vi "niFPGA BW CU Order 4 (32-bit).vi"(0 "filter state in":T1, 1 "reset":bool, 5 "input data":i32, 7 "accumulator in":fxp<+/-,36,32>, 9 "adder in":fxp<+/-,34,34>, 11 "iteration":u8, 12 "In shift":i8=-1, 13 "lowpass?":bool) -> (4 "filter state out":T1, 6 "state to multiply":i32, 8 "accumulator out":fxp<+/-,36,32> format="%.14g", 10 "adder out":fxp<+/-,34,34>, 15 "terminate":bool)   [LabVIEW 2017]
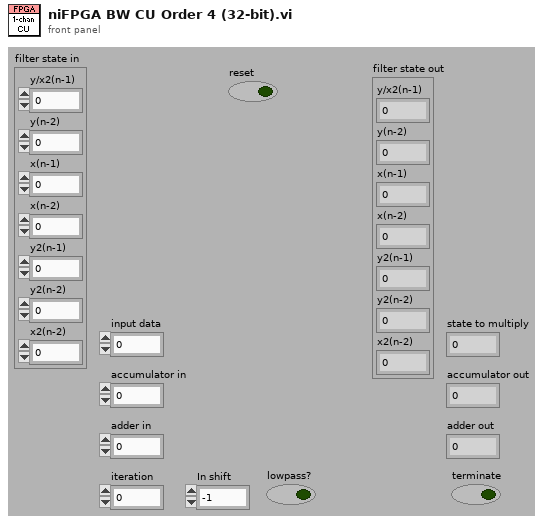
[diagram p1: front panel]
types:
  T1 = cluster{"y/x2(n-1)":i32, "y(n-2)":i32, "x(n-1)":i32, "x(n-2)":i32, "y2(n-1)":i32, "y2(n-2)":i32, "x2(n-2)":i32}
  T2 = cluster{"y(n)=x(n) 2":i32, "y(n-2)":i32, "x(n-1)":i32, "x(n-2)":i32, "y(n-1) 2":i32, "y(n-2) 2":i32, "x(n-2) 2":i32}
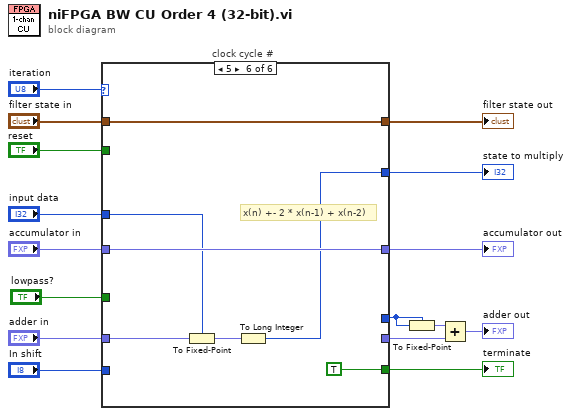
[diagram p0: block diagram]
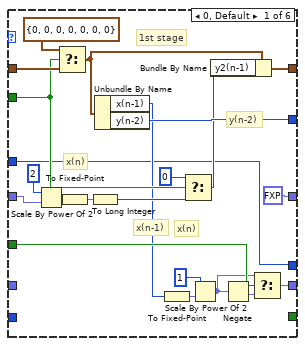
[diagram p2: hidden frame]
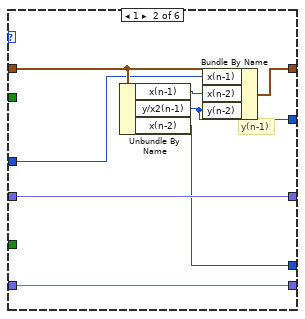
[diagram p3: hidden frame]
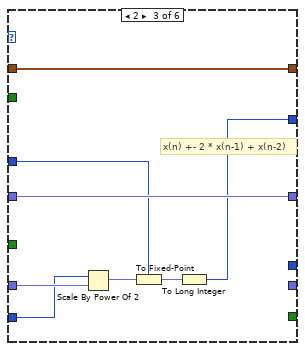
[diagram p4: hidden frame]
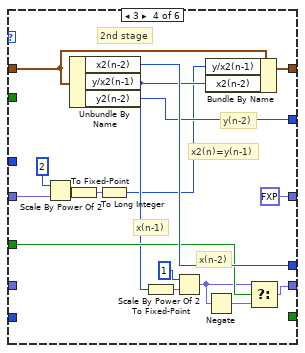
[diagram p5: hidden frame]
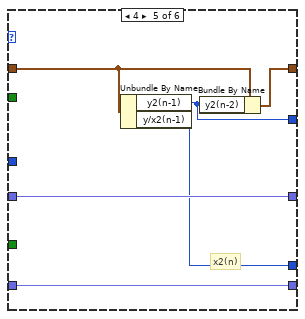
[diagram p6: hidden frame]
diagram:
  n1 = case "clock cycle #" shown="5" "iteration" {
    tunnel: [w38 w42 w53 w71 w73 w82] -> w3
    tunnel: "input data" -> [w17 w41 w47 _ _ w78]
    tunnel: [w28 w46 _ w61 w77 _] -> w10
    tunnel: "adder in" -> [_ w46 w50 _ w77 w80]
    tunnel: [w36 w44 w49 w69 w75 w81] -> w12
    tunnel: [w17 w39 _ w70 w72 _] -> w2
    tunnel: [fxp<+/-,36,32> 0.0 ("Numeric") w45 w54 fxp<+/-,36,32> 0.0 ("accumulator in") w76 w83] -> w11
    tunnel: [_ _ _ _ _ TRUE] -> w9
    tunnel: "reset" -> [w31 _ _ _ _ _]
    tunnel: "accumulator in" -> [w25 w45 w54 w60 w76 w83]
    tunnel: "filter state in" -> [w32 w43 w53 w66 w74 w82]
    tunnel: "In shift" -> [_ _ w48 _ _ _]
    tunnel: "lowpass?" -> [w29 _ _ w67 _ _]
    frame 0, Default {
      # "1st stage"
      # "x(n)"
      # "x(n)"
      # "x(n-1)"
      # "y(n-2)"
      n2 = Scale By Power Of 2(n=2, x=w25) -> (x*2^n=w26:fxp<+/-,36,32>)
      n3 = Select(t=T2 {"y(n)=x(n) 2"=0, "y(n-2)"=0, "x(n-1)"=0, "x(n-2)"=0, "y(n-1) 2"=0, "y(n-2) 2"=0, "x(n-2) 2"=0} ("output cluster"), s=w31, f=w32) -> (s? t:f=w34:T1)
      n4 = To Fixed-Point(number=w26) -> (fixed-point=w27:fxp<+/-,32,32>)  [unwired: 1 out]
      n5 = To Long Integer(number=w27) -> (32bit integer=w23:i32)
      n6 = Unbundle By Name(w34) -> ("x(n-1)"=w19:i32, "y(n-2)"=w36:i32)
      n7 = To Fixed-Point(number=w19) -> (fixed-point=w21:fxp<+/-,33,33>)  [unwired: 1 out]
      n8 = Select(t=0, s=w31, f=w23) -> (s? t:f=w22:i32)
      n9 = Scale By Power Of 2(n=1, x=w21) -> (x*2^n=w18:fxp<+/-,33,33>)
      n10 = Bundle By Name(cluster=w34, "y2(n-1)"=w22) -> (w38:T1)
      n11 = Negate(x=w18) -> (-x=w30:fxp<+/-,34,34>)
      n12 = Select(t=w18, s=w29, f=w30) -> (s? t:f=w28:fxp<+/-,34,34>)
    }
    frame 1 {
      # "y(n-1)"
      n13 = Unbundle By Name(w43) -> ("x(n-1)"=w40:i32, "y/x2(n-1)"=w44:i32, "x(n-2)"=w39:i32)
      n14 = Bundle By Name(cluster=w43, "x(n-1)"=w41, "x(n-2)"=w40, "y(n-2)"=w44) -> (w42:T1)
    }
    frame 2 {
      # "x(n) +- 2 * x(n-1) + x(n-2)"
      n15 = Scale By Power Of 2(n=w48, x=w50) -> (x*2^n=w52:fxp<+/-,34,34>)
      n16 = To Fixed-Point(fixed-point type=w47, number=w52) -> (fixed-point=w51:fxp<+/-,32,32>)
      n17 = To Long Integer(number=w51) -> (32bit integer=w49:i32)
    }
    frame 3 {
      # "x2(n)=y(n-1)"
      # "2nd stage"
      # "x(n-2)"
      # "x(n-1)"
      # "y(n-2)"
      n18 = Scale By Power Of 2(n=2, x=w60) -> (x*2^n=w58:fxp<+/-,36,32>)
      n19 = To Fixed-Point(number=w58) -> (fixed-point=w57:fxp<+/-,32,32>)  [unwired: 1 out]
      n20 = Unbundle By Name(w66) -> ("x2(n-2)"=w70:i32, "y/x2(n-1)"=w63:i32, "y2(n-2)"=w69:i32)
      n21 = To Long Integer(number=w57) -> (32bit integer=w56:i32)
      n22 = To Fixed-Point(number=w63) -> (fixed-point=w65:fxp<+/-,33,33>)  [unwired: 1 out]
      n23 = Scale By Power Of 2(n=1, x=w65) -> (x*2^n=w62:fxp<+/-,33,33>)
      n24 = Bundle By Name(cluster=w66, "y/x2(n-1)"=w56, "x2(n-2)"=w63) -> (w71:T1)
      n25 = Negate(x=w62) -> (-x=w68:fxp<+/-,34,34>)
      n26 = Select(t=w62, s=w67, f=w68) -> (s? t:f=w61:fxp<+/-,34,34>)
    }
    frame 4 {
      # "x2(n)"
      n27 = Unbundle By Name(w74) -> ("y2(n-1)"=w75:i32, "y/x2(n-1)"=w72:i32)
      n28 = Bundle By Name(cluster=w74, "y2(n-2)"=w75) -> (w73:T1)
    }
    frame 5 {
      # "x(n) +- 2 * x(n-1) + x(n-2)"
      n29 = To Fixed-Point(fixed-point type=w78, number=w80) -> (fixed-point=w79:fxp<+/-,32,32>)
      n30 = To Long Integer(number=w79) -> (32bit integer=w81:i32)
    }
  }
  "state to multiply" <- w12
  "terminate" <- w9
  "accumulator out" <- w11
  "filter state out" <- w3
  n31 = To Fixed-Point(fixed-point type=w2, number=w2) -> (fixed-point=w1:fxp<+/-,32,32>)
  n32 = Add(x=w1, y=w10) -> (x+y=→"adder out":fxp<+/-,34,34>)
